vi "Query Multi Eval Meas ES Flatness Limit Check Results.vi"(8 "error in (no error)":errorcluster, 9 "Result Type (Current)":i32(ring) items=["Current", "Average", "Extreme"], 10 "Instance (1)":T2=1, 11 "VISA resource name":refnum<visa-resource-name>) -> (0 "error out":errorcluster, 1 "ES Flatness Limit Check Results":T1 {"Out Of Tolerance" format="%^.3e"}, 2 "Reliability":i32, 3 "VISA resource name out":refnum<visa-resource-name>)   [LabVIEW 2015, in "Rohde&Schwarz CMXP NR FR2 Measurement.lvlib"]
doc: "Starts a new single shot measurement and returns the multi eval measurement ES Flatness results.\n\nAttributes:\nRSCMXPNRFR2M_ATTR_QUERY_MULTI_EVAL_MEASUREMENT_ESF_AVERAGE_LIMIT_CHECK_RESULTS\nRSCMXPNRFR2M_ATTR_QUERY_MULTI_EVAL_MEASUREMENT_ESF_CURRENT_LIMIT_CHECK_RESULTS\nRSCMXPNRFR2M_ATTR_QUERY_MULTI_EVAL_MEASUREMENT_ESF_EXTREME_LIMIT_CHECK_RESULTS\n\nRemote-control commands:\nCALCulate:NRMMw:MEAS<i>:MEValuation:ESFLatness:AVERage?\nCALCulate:NRMMw:MEAS<i>:MEValuation:ESFLatness:CURRent?\nCALCulate:NRMMw:MEAS<i>:MEValuation:ESFLatness:EXTReme?"
uses:
  <instrlib>/Rohde&Schwarz CMXP NR FR2 Measurement/Rohde&Schwarz CMXP NR FR2 Measurement.lvlib
  <instrlib>/Rohde&Schwarz CMXP NR FR2 Measurement/Private/_Instance.ctl
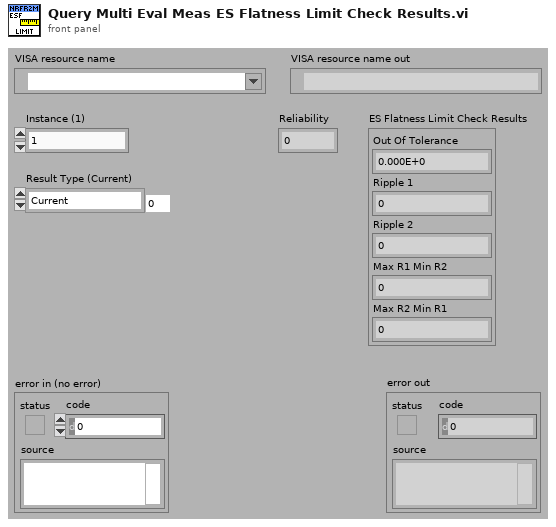
[diagram p1: front panel]
types:
  T1 = cluster{"Out Of Tolerance":dbl, "Ripple 1":i32, "Ripple 2":i32, "Max R1 Min R2":i32, "Max R2 Min R1":i32}
  T2 = typedef "Rohde&Schwarz CMXP NR FR2 Measurement.lvlib/_Instance.ctl" = i32
  T3 = cluster{"Out Of Tolerance":dbl, "Val 1":i32, "Val 2":i32, "Val 3":i32, "Val 4":i32}
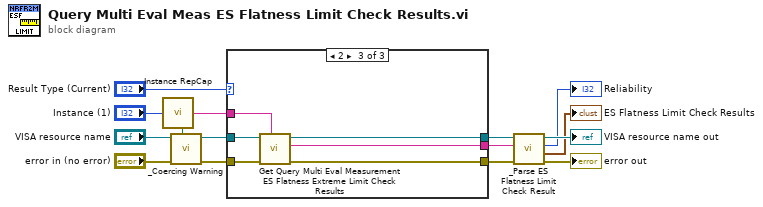
[diagram p0: block diagram]
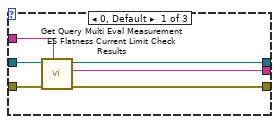
[diagram p2: hidden frame]
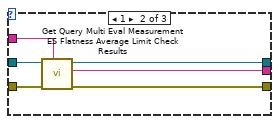
[diagram p3: hidden frame]
diagram:
  n1 = call <instrlib>:"Instance RepCap.vi"("Instance In"="Instance (1)") -> ("In Range?"=w3:bool, "RepCap Identifier Out"=w14:string)  [unwired: 1 in]
  n2 = call <instrlib>:"_Coercing Warning.vi"("In Range?"=w3, "error in (no error)"="error in (no error)", "VISA resource name"="VISA resource name") -> ("error out"=w4:errorcluster, "VISA resource name out"=w5:refnum<visa-resource-name>)  [unwired: 7 in]
  n3 = case shown="2" "Result Type (Current)" {
    tunnel: w4 -> [w21 w27 w33]
    tunnel: w5 -> [w20 w26 w32]
    tunnel: [w19 w25 w31] -> w12
    tunnel: [w18 w24 w30] -> w11
    tunnel: w14 -> [w17 w23 w29]
    tunnel: [w16 w22 w28] -> w13
    frame 0, Default {
      n4 = call "Get Query Multi Eval Measurement ES Flatness Current Limit Check Results"("Repeated Capabilities"=w17, "error in (no error)"=w21, "instrument handle"=w20) -> ("error out"=w19:errorcluster, "Query Multi Eval Measurement ES Flatness Current Limit Check Results"=w16:string, "instrument handle out"=w18:refnum<visa-resource-name>)  [unwired: 6 in]
    }
    frame 1 {
      n5 = call "Get Query Multi Eval Measurement ES Flatness Average Limit Check Results"("Repeated Capabilities"=w23, "error in (no error)"=w27, "instrument handle"=w26) -> ("error out"=w25:errorcluster, "Query Multi Eval Measurement ES Flatness Average Limit Check Results"=w22:string, "instrument handle out"=w24:refnum<visa-resource-name>)  [unwired: 6 in]
    }
    frame 2 {
      n6 = call "Get Query Multi Eval Measurement ES Flatness Extreme Limit Check Results"("Repeated Capabilities"=w29, "error in (no error)"=w33, "instrument handle"=w32) -> ("error out"=w31:errorcluster, "Query Multi Eval Measurement ES Flatness Extreme Limit Check Results"=w28:string, "instrument handle out"=w30:refnum<visa-resource-name>)  [unwired: 6 in]
    }
  }
  n7 = call <instrlib>:"_Parse ES Flatness Limit Check Result.vi"("error in (no error)"=w12, "Input String"=w13, "VISA resource name"=w11) -> ("error out"=→"error out":errorcluster, "Result"=→"ES Flatness Limit Check Results":T3, "Reliability"=→"Reliability":i32, "VISA resource name out"=→"VISA resource name out":refnum<visa-resource-name>)  [unwired: 5 in]
